vi "Route GPIO Lines.vi"(0 "user gpio bank in":T3, 5 "gpio routes":i8[](array[numeric])=[0, 0, 0, 0, 0, 0, 0, 0, 0, 0, 0, 0, 0, 0, 0, 0, 0, 0, 0, 0, 0, 0, 0, 0, 0, 0, 0, 0, 0, 0, 0, 0, 0, 0, 0, 0, 0, 0, 0, 0, 0, 0, 0, 0, 0, 0, 0, 0, 0, 0, 0, 0, 0, 0, 0, 0, 0, 0, 0, 0, 0, 0, 0, 0, 0, 0, 0, 0, 0, 0, 0, 0, 0, 0, 0, 0, 0, 0, 0, 0, 0, 0, 0, 0, 0, 0, 0, 0, 0, 0, 0, 0, 0, 0, 0, 0], 11 "override gpio bank ouptut configs":T1[](array[typedef])) -> (4 "user gpio bank out":T3)   [LabVIEW 2020, in "GettingStarted_Common_148X_FPGA.lvlib"]
uses:
  GettingStarted_Common_148X_FPGA.lvlib
  Types/GPIO User Bank.ctl
  Types/GPIO Bank Output Configuration.ctl
  <instrlib>/FlexRIO/CSI-2/v2/FPGA/Types/GPIO Bank.ctl
  Types/SerDes Identifier.ctl
  <instrlib>/FlexRIO/CSI-2/v2/FPGA/NI CSI-2 API FPGA v2.lvlib
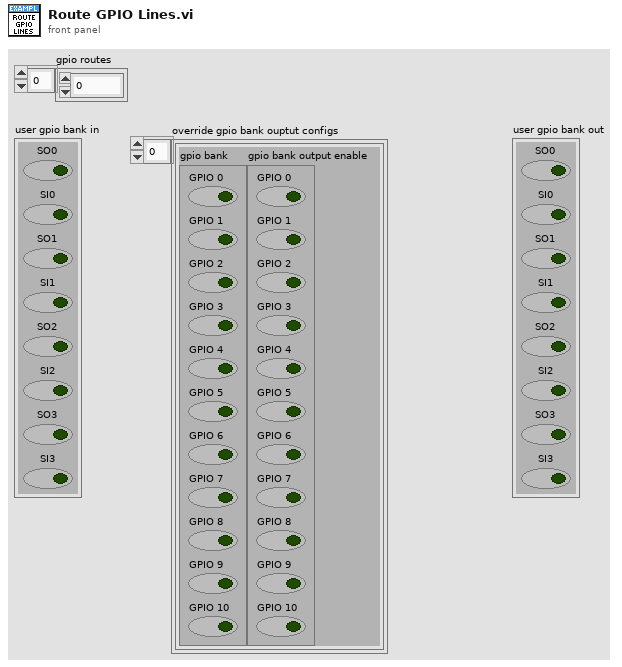
[diagram p1: front panel]
types:
  T1 = typedef "GettingStarted_Common_148X_FPGA.lvlib/GPIO Bank Output Configuration.ctl" = cluster{"gpio bank":T2, "gpio bank output enable":T2}
  T2 = typedef "NI CSI-2 API FPGA v2.lvlib/GPIO Bank.ctl" = cluster{"GPIO 0":bool, "GPIO 1":bool, "GPIO 2":bool, "GPIO 3":bool, "GPIO 4":bool, "GPIO 5":bool, "GPIO 6":bool, "GPIO 7":bool, "GPIO 8":bool, "GPIO 9":bool, "GPIO 10":bool}
  T3 = typedef "GettingStarted_Common_148X_FPGA.lvlib/GPIO User Bank.ctl" = cluster{"SO0":bool, "SI0":bool, "SO1":bool, "SI1":bool, "SO2":bool, "SI2":bool, "SO3":bool, "SI3":bool}
  T4 = typedef "GettingStarted_Common_148X_FPGA.lvlib/SerDes Identifier.ctl" = enum8{"None", "SI 0 Deserializer", "SI 1 Deserializer", "SI 2 Deserializer", "SI 3 Deserializer", "SI 4 Deserializer", "SI 5 Deserializer", "SI 6 Deserializer", "SI 7 Deserializer", "SO 0 Serializer", "SO 1 Serializer", "SO 2 Serializer", "SO 3 Serializer", "SO 4 Serializer", "SO 5 Serializer", "SO 6 Serializer", "SO 7 Serializer", "SI 0 SI 1 Deserializer", "SI 2 SI 3 Deserializer", "SI 4 SI 5 Deserializer", "SI 6 SI 7 Deserializer"}
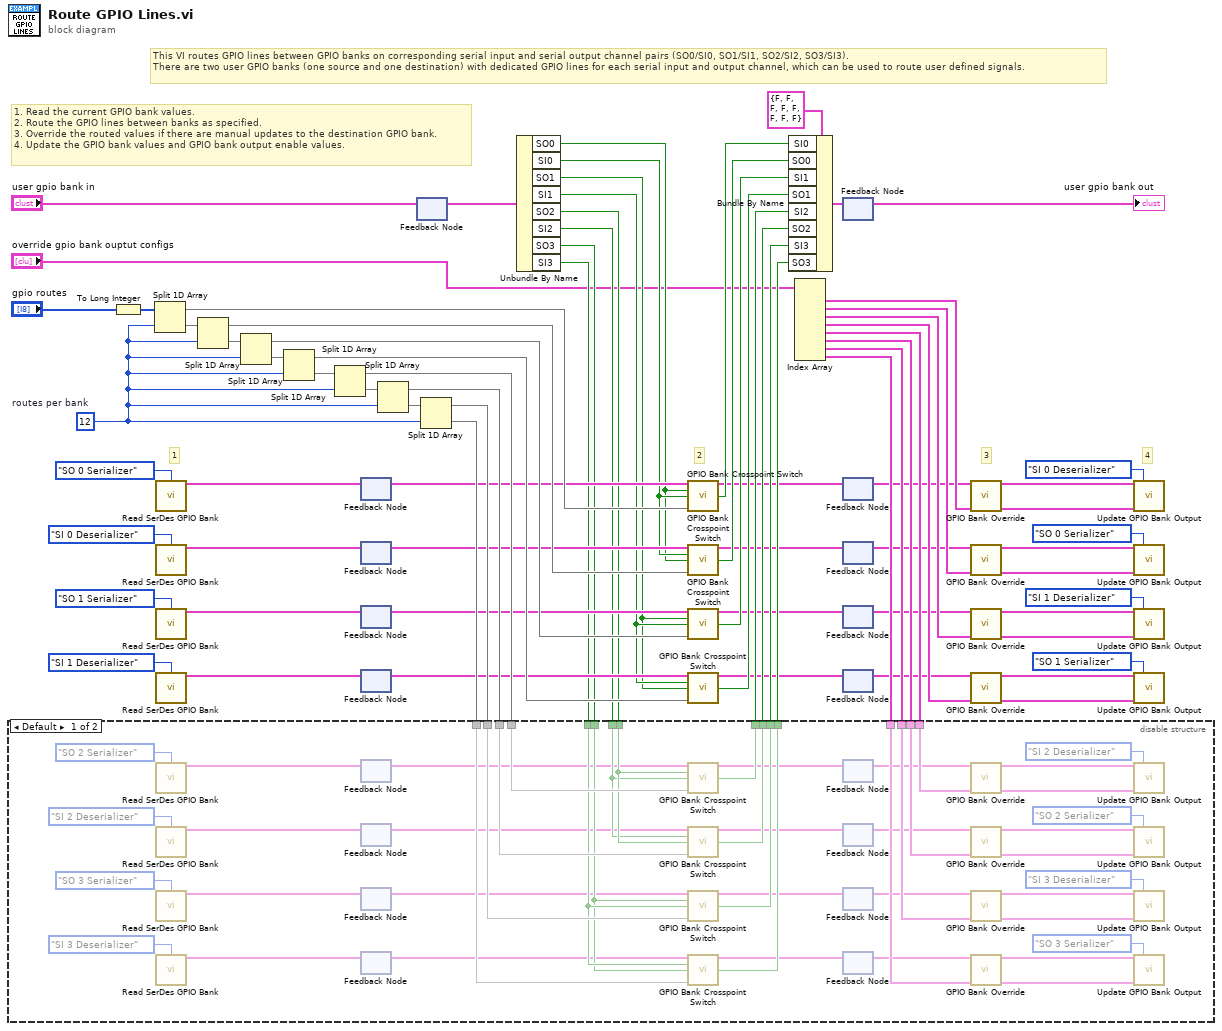
[diagram p0: block diagram]
diagram:
  w68 = 12  # routes per bank
  # "1. Read the current GPIO bank values.\n2. Route the GPIO lines between banks as specified.\n3. Override the routed values if there are manual updates to the destination GPIO bank.\n4. Update the GPIO bank values and GPIO bank output enable values."
  # "4"
  # "3"
  # "2"
  # "1"
  # "This VI routes GPIO lines between GPIO banks on corresponding serial input and serial output channel pairs (SO0/SI0, SO1/SI1, SO2/SI2, SO3/SI3). \nThere are two user GPIO banks (one source and one destination) with dedicated GPIO lines for each serial input and output channel, which can be used to route user defined signals."
  n1 = To Long Integer(number="gpio routes") -> (32bit integer=w75:i32[])
  n2 = Split 1D Array(array=w75, index=w68) -> (first subarray=w61:i32[], second subarray=w74:i32[])
  n3 = call "Read SerDes GPIO Bank.vi"("serdes id"=SerDes_Identifier."SO 0 Serializer") -> ("gpio bank input"=w52:T2)  [unwired: 13 in, 1 out]
  n4 = call "Read SerDes GPIO Bank.vi"("serdes id"=SerDes_Identifier."SI 0 Deserializer") -> ("gpio bank input"=w53:T2)  [unwired: 13 in, 1 out]
  n5 = call "Read SerDes GPIO Bank.vi"("serdes id"=SerDes_Identifier."SO 1 Serializer") -> ("gpio bank input"=w51:T2)  [unwired: 13 in, 1 out]
  n6 = call "Read SerDes GPIO Bank.vi"("serdes id"=SerDes_Identifier."SI 1 Deserializer") -> ("gpio bank input"=w50:T2)  [unwired: 13 in, 1 out]
  n7 = Split 1D Array(array=w74, index=w68) -> (first subarray=w60:i32[], second subarray=w73:i32[])
  n8 = Split 1D Array(array=w73, index=w68) -> (first subarray=w59:i32[], second subarray=w70:i32[])
  n9 = Split 1D Array(array=w70, index=w68) -> (first subarray=w58:i32[], second subarray=w71:i32[])
  n10 = Split 1D Array(array=w71, index=w68) -> (first subarray=w57:i32[], second subarray=w72:i32[])
  n11 = feedback #1() -> (w29:T2)  [unwired: 1 in]
  n12 = feedback-in #1(w52) -> ()
  n13 = feedback #2() -> (w28:T2)  [unwired: 1 in]
  n14 = feedback-in #2(w53) -> ()
  n15 = feedback #3() -> (w27:T2)  [unwired: 1 in]
  n16 = feedback-in #3(w51) -> ()
  n17 = feedback #4() -> (w26:T2)  [unwired: 1 in]
  n18 = feedback-in #4(w50) -> ()
  n19 = Split 1D Array(array=w72, index=w68) -> (first subarray=w56:i32[], second subarray=w69:i32[])
  n20 = feedback #5() -> (w78:T3)  [unwired: 1 in]
  n21 = feedback-in #5("user gpio bank in") -> ()
  n22 = Split 1D Array(array=w69, index=w68) -> (first subarray=w55:i32[], second subarray=w54:i32[])
  n23 = Unbundle By Name(w78) -> ("SO0"=w18:bool, "SI0"=w19:bool, "SO1"=w20:bool, "SI1"=w21:bool, "SO2"=w23:bool, "SI2"=w22:bool, "SO3"=w24:bool, "SI3"=w25:bool)
  n24 = call "GPIO Bank Crosspoint Switch.vi"("source gpio bank in"=w29, "source user gpio in"=w18, "destination user gpio in"=w19, "gpio bank routing"=w61) -> ("destination gpio bank output config"=w30:T1, "destination user gpio out"=w31:bool)  [unwired: 10 in]
  n25 = call "GPIO Bank Crosspoint Switch.vi"("source gpio bank in"=w28, "source user gpio in"=w19, "destination user gpio in"=w18, "gpio bank routing"=w60) -> ("destination gpio bank output config"=w32:T1, "destination user gpio out"=w33:bool)  [unwired: 10 in]
  n26 = call "GPIO Bank Crosspoint Switch.vi"("source gpio bank in"=w27, "source user gpio in"=w20, "destination user gpio in"=w21, "gpio bank routing"=w59) -> ("destination gpio bank output config"=w34:T1, "destination user gpio out"=w35:bool)  [unwired: 10 in]
  n27 = call "GPIO Bank Crosspoint Switch.vi"("source gpio bank in"=w26, "source user gpio in"=w21, "destination user gpio in"=w20, "gpio bank routing"=w58) -> ("destination gpio bank output config"=w36:T1, "destination user gpio out"=w37:bool)  [unwired: 10 in]
  n28 = Index Array(array="override gpio bank ouptut configs") -> (element #1=w49:T1, element #2=w48:T1, element #3=w47:T1, element #4=w46:T1, element #5=w45:T1, element #6=w44:T1, element #7=w43:T1, element #8=w42:T1)  [unwired: 8 in]
  n29 = disable-structure shown="Default" {
    disable-tunnel: w57 -> [w127 _]
    disable-tunnel: w56 -> [w126 _]
    disable-tunnel: w55 -> [w125 _]
    disable-tunnel: w54 -> [w124 _]
    disable-tunnel: w45 -> [w123 _]
    disable-tunnel: w44 -> [w122 _]
    disable-tunnel: w43 -> [w121 _]
    disable-tunnel: w42 -> [w120 _]
    disable-tunnel: [w119 _] -> w41
    disable-tunnel: [w118 _] -> w40
    disable-tunnel: [w117 _] -> w39
    disable-tunnel: [w116 _] -> w38
    disable-tunnel: w25 -> [w115 _]
    disable-tunnel: w24 -> [w114 _]
    disable-tunnel: w23 -> [w113 _]
    disable-tunnel: w22 -> [w112 _]
    frame condition #0 {
      n30 = call "Read SerDes GPIO Bank.vi"("serdes id"=SerDes_Identifier."SO 2 Serializer") -> ("gpio bank input"=w105:T2)  [unwired: 13 in, 1 out]
      n31 = call "Read SerDes GPIO Bank.vi"("serdes id"=SerDes_Identifier."SI 2 Deserializer") -> ("gpio bank input"=w104:T2)  [unwired: 13 in, 1 out]
      n32 = call "Read SerDes GPIO Bank.vi"("serdes id"=SerDes_Identifier."SO 3 Serializer") -> ("gpio bank input"=w107:T2)  [unwired: 13 in, 1 out]
      n33 = call "Read SerDes GPIO Bank.vi"("serdes id"=SerDes_Identifier."SI 3 Deserializer") -> ("gpio bank input"=w106:T2)  [unwired: 13 in, 1 out]
      n34 = feedback #6() -> (w99:T2)  [unwired: 1 in]
      n35 = feedback-in #6(w105) -> ()
      n36 = feedback #7() -> (w98:T2)  [unwired: 1 in]
      n37 = feedback-in #7(w104) -> ()
      n38 = feedback #8() -> (w97:T2)  [unwired: 1 in]
      n39 = feedback-in #8(w107) -> ()
      n40 = feedback #9() -> (w96:T2)  [unwired: 1 in]
      n41 = feedback-in #9(w106) -> ()
      n42 = call "GPIO Bank Crosspoint Switch.vi"("source gpio bank in"=w99, "source user gpio in"=w113, "destination user gpio in"=w112, "gpio bank routing"=w127) -> ("destination gpio bank output config"=w100:T1, "destination user gpio out"=w116:bool)  [unwired: 10 in]
      n43 = call "GPIO Bank Crosspoint Switch.vi"("source gpio bank in"=w98, "source user gpio in"=w112, "destination user gpio in"=w113, "gpio bank routing"=w126) -> ("destination gpio bank output config"=w101:T1, "destination user gpio out"=w117:bool)  [unwired: 10 in]
      n44 = call "GPIO Bank Crosspoint Switch.vi"("source gpio bank in"=w97, "source user gpio in"=w114, "destination user gpio in"=w115, "gpio bank routing"=w125) -> ("destination gpio bank output config"=w102:T1, "destination user gpio out"=w118:bool)  [unwired: 10 in]
      n45 = call "GPIO Bank Crosspoint Switch.vi"("source gpio bank in"=w96, "source user gpio in"=w115, "destination user gpio in"=w114, "gpio bank routing"=w124) -> ("destination gpio bank output config"=w103:T1, "destination user gpio out"=w119:bool)  [unwired: 10 in]
      n46 = feedback #10() -> (w95:T1)  [unwired: 1 in]
      n47 = feedback-in #10(w100) -> ()
      n48 = feedback #11() -> (w94:T1)  [unwired: 1 in]
      n49 = feedback-in #11(w101) -> ()
      n50 = feedback #12() -> (w93:T1)  [unwired: 1 in]
      n51 = feedback-in #12(w102) -> ()
      n52 = feedback #13() -> (w92:T1)  [unwired: 1 in]
      n53 = feedback-in #13(w103) -> ()
      n54 = call "GPIO Bank Override.vi"("gpio bank output config"=w95, "override gpio bank output config"=w123) -> ("gpio bank"=w89:T2, "gpio bank output enable"=w83:T2)  [unwired: 12 in]
      n55 = call "GPIO Bank Override.vi"("gpio bank output config"=w94, "override gpio bank output config"=w122) -> ("gpio bank"=w88:T2, "gpio bank output enable"=w82:T2)  [unwired: 12 in]
      n56 = call "GPIO Bank Override.vi"("gpio bank output config"=w93, "override gpio bank output config"=w121) -> ("gpio bank"=w87:T2, "gpio bank output enable"=w81:T2)  [unwired: 12 in]
      n57 = call "GPIO Bank Override.vi"("gpio bank output config"=w92, "override gpio bank output config"=w120) -> ("gpio bank"=w91:T2, "gpio bank output enable"=w80:T2)  [unwired: 12 in]
      n58 = call "Update GPIO Bank Output.vi"("gpio bank"=w89, "gpio bank serdes id"=SerDes_Identifier."SI 2 Deserializer" ("serdes id"), "gpio bank output enable"=w83) -> ()  [unwired: 12 in, 1 out]
      n59 = call "Update GPIO Bank Output.vi"("gpio bank"=w88, "gpio bank serdes id"=SerDes_Identifier."SO 2 Serializer" ("serdes id"), "gpio bank output enable"=w82) -> ()  [unwired: 12 in, 1 out]
      n60 = call "Update GPIO Bank Output.vi"("gpio bank"=w87, "gpio bank serdes id"=SerDes_Identifier."SI 3 Deserializer" ("serdes id"), "gpio bank output enable"=w81) -> ()  [unwired: 12 in, 1 out]
      n61 = call "Update GPIO Bank Output.vi"("gpio bank"=w91, "gpio bank serdes id"=SerDes_Identifier."SO 3 Serializer" ("serdes id"), "gpio bank output enable"=w80) -> ()  [unwired: 12 in, 1 out]
    }
    frame condition #1 (active) {
    }
  }
  n62 = Bundle By Name(cluster=T3 {"SO0"=FALSE, "SI0"=FALSE, "SO1"=FALSE, "SI1"=FALSE, "SO2"=FALSE, "SI2"=FALSE, "SO3"=FALSE, "SI3"=FALSE} ("user gpio bank"), "SI0"=w31, "SO0"=w33, "SI1"=w35, "SO1"=w37, "SI2"=w38, "SO2"=w39, "SI3"=w40, "SO3"=w41) -> (w77:T3)
  n63 = feedback #14() -> (→"user gpio bank out":T3)  [unwired: 1 in]
  n64 = feedback-in #14(w77) -> ()
  n65 = feedback #15() -> (w16:T1)  [unwired: 1 in]
  n66 = feedback-in #15(w30) -> ()
  n67 = feedback #16() -> (w15:T1)  [unwired: 1 in]
  n68 = feedback-in #16(w32) -> ()
  n69 = feedback #17() -> (w14:T1)  [unwired: 1 in]
  n70 = feedback-in #17(w34) -> ()
  n71 = feedback #18() -> (w13:T1)  [unwired: 1 in]
  n72 = feedback-in #18(w36) -> ()
  n73 = call "GPIO Bank Override.vi"("gpio bank output config"=w16, "override gpio bank output config"=w49) -> ("gpio bank"=w12:T2, "gpio bank output enable"=w4:T2)  [unwired: 12 in]
  n74 = call "GPIO Bank Override.vi"("gpio bank output config"=w15, "override gpio bank output config"=w48) -> ("gpio bank"=w11:T2, "gpio bank output enable"=w3:T2)  [unwired: 12 in]
  n75 = call "GPIO Bank Override.vi"("gpio bank output config"=w14, "override gpio bank output config"=w47) -> ("gpio bank"=w10:T2, "gpio bank output enable"=w2:T2)  [unwired: 12 in]
  n76 = call "GPIO Bank Override.vi"("gpio bank output config"=w13, "override gpio bank output config"=w46) -> ("gpio bank"=w9:T2, "gpio bank output enable"=w1:T2)  [unwired: 12 in]
  n77 = call "Update GPIO Bank Output.vi"("gpio bank"=w12, "gpio bank serdes id"=SerDes_Identifier."SI 0 Deserializer" ("serdes id"), "gpio bank output enable"=w4) -> ()  [unwired: 12 in, 1 out]
  n78 = call "Update GPIO Bank Output.vi"("gpio bank"=w11, "gpio bank serdes id"=SerDes_Identifier."SO 0 Serializer" ("serdes id"), "gpio bank output enable"=w3) -> ()  [unwired: 12 in, 1 out]
  n79 = call "Update GPIO Bank Output.vi"("gpio bank"=w10, "gpio bank serdes id"=SerDes_Identifier."SI 1 Deserializer" ("serdes id"), "gpio bank output enable"=w2) -> ()  [unwired: 12 in, 1 out]
  n80 = call "Update GPIO Bank Output.vi"("gpio bank"=w9, "gpio bank serdes id"=SerDes_Identifier."SO 1 Serializer" ("serdes id"), "gpio bank output enable"=w1) -> ()  [unwired: 12 in, 1 out]
